vi "about GUI.vi"(8 "error in (no error)":errorcluster) -> (0 "error out":errorcluster)   [LabVIEW 2020, in "main.lvlib"]
uses:
  main.lvlib
  PTRL/GUI_tools/GUI_tools.lvlib
panel:
  out "about message":string
  in  "bottom_right":u32(colorbox)=16764108
  in  "top_left":u32(colorbox)=13434847
  # "Visible to user"
  # "Knight Tour"
  # "Resources\n1. https://en.wikipedia.org/wiki/Knight%27s_tour\n2. http://www.behnel.de/knight.html\n3. http://www.axel-conrad.de/springer/springer.html\n4. https://oeis.org/A165134 \n5. https://oeis.org/A165134/a165134.txt"
  # "Invisible to user"
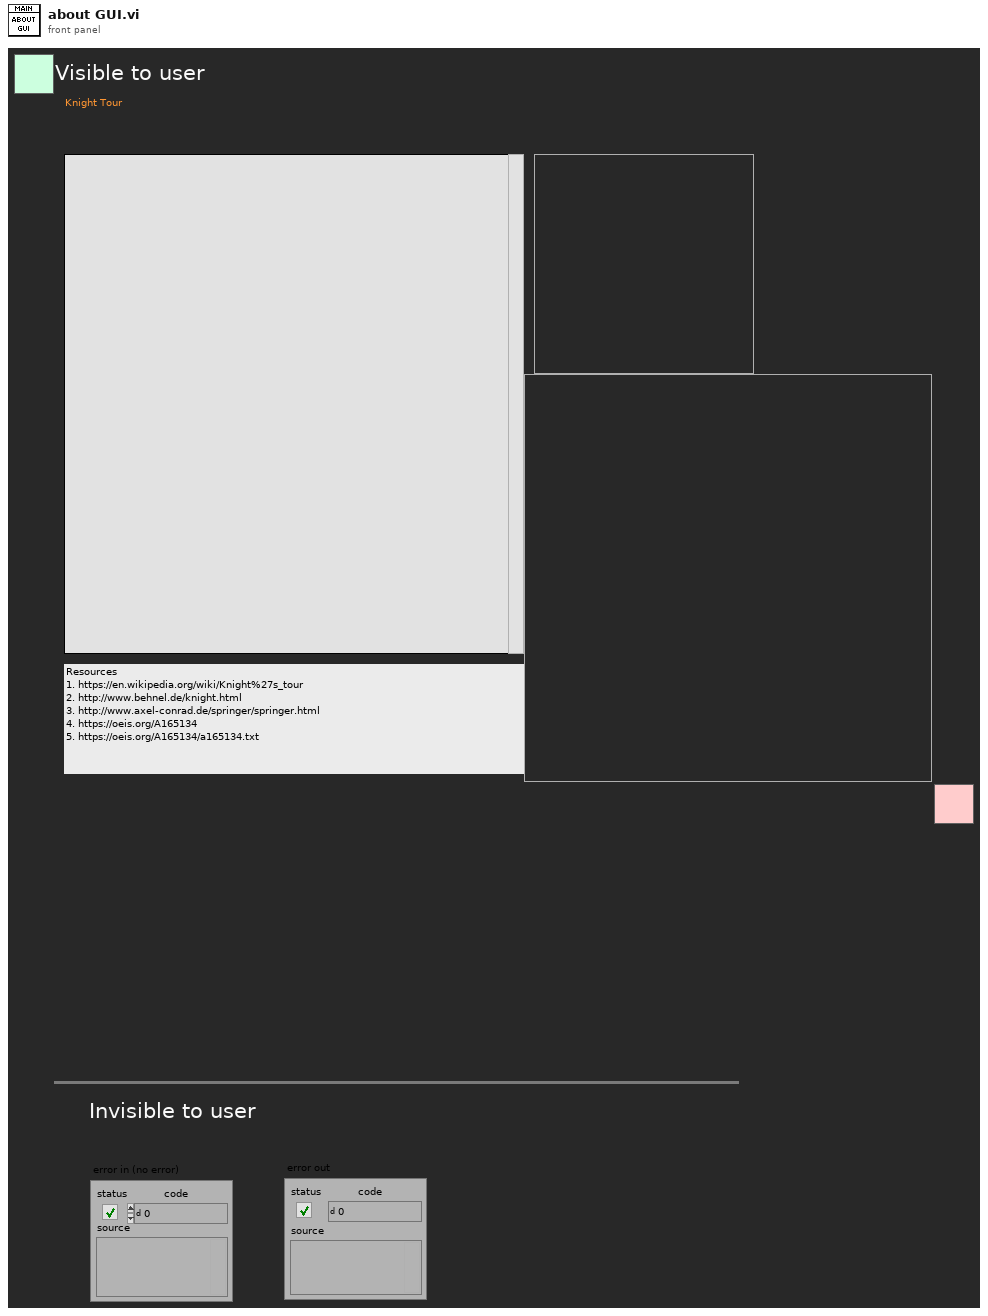
[diagram p1: front panel]
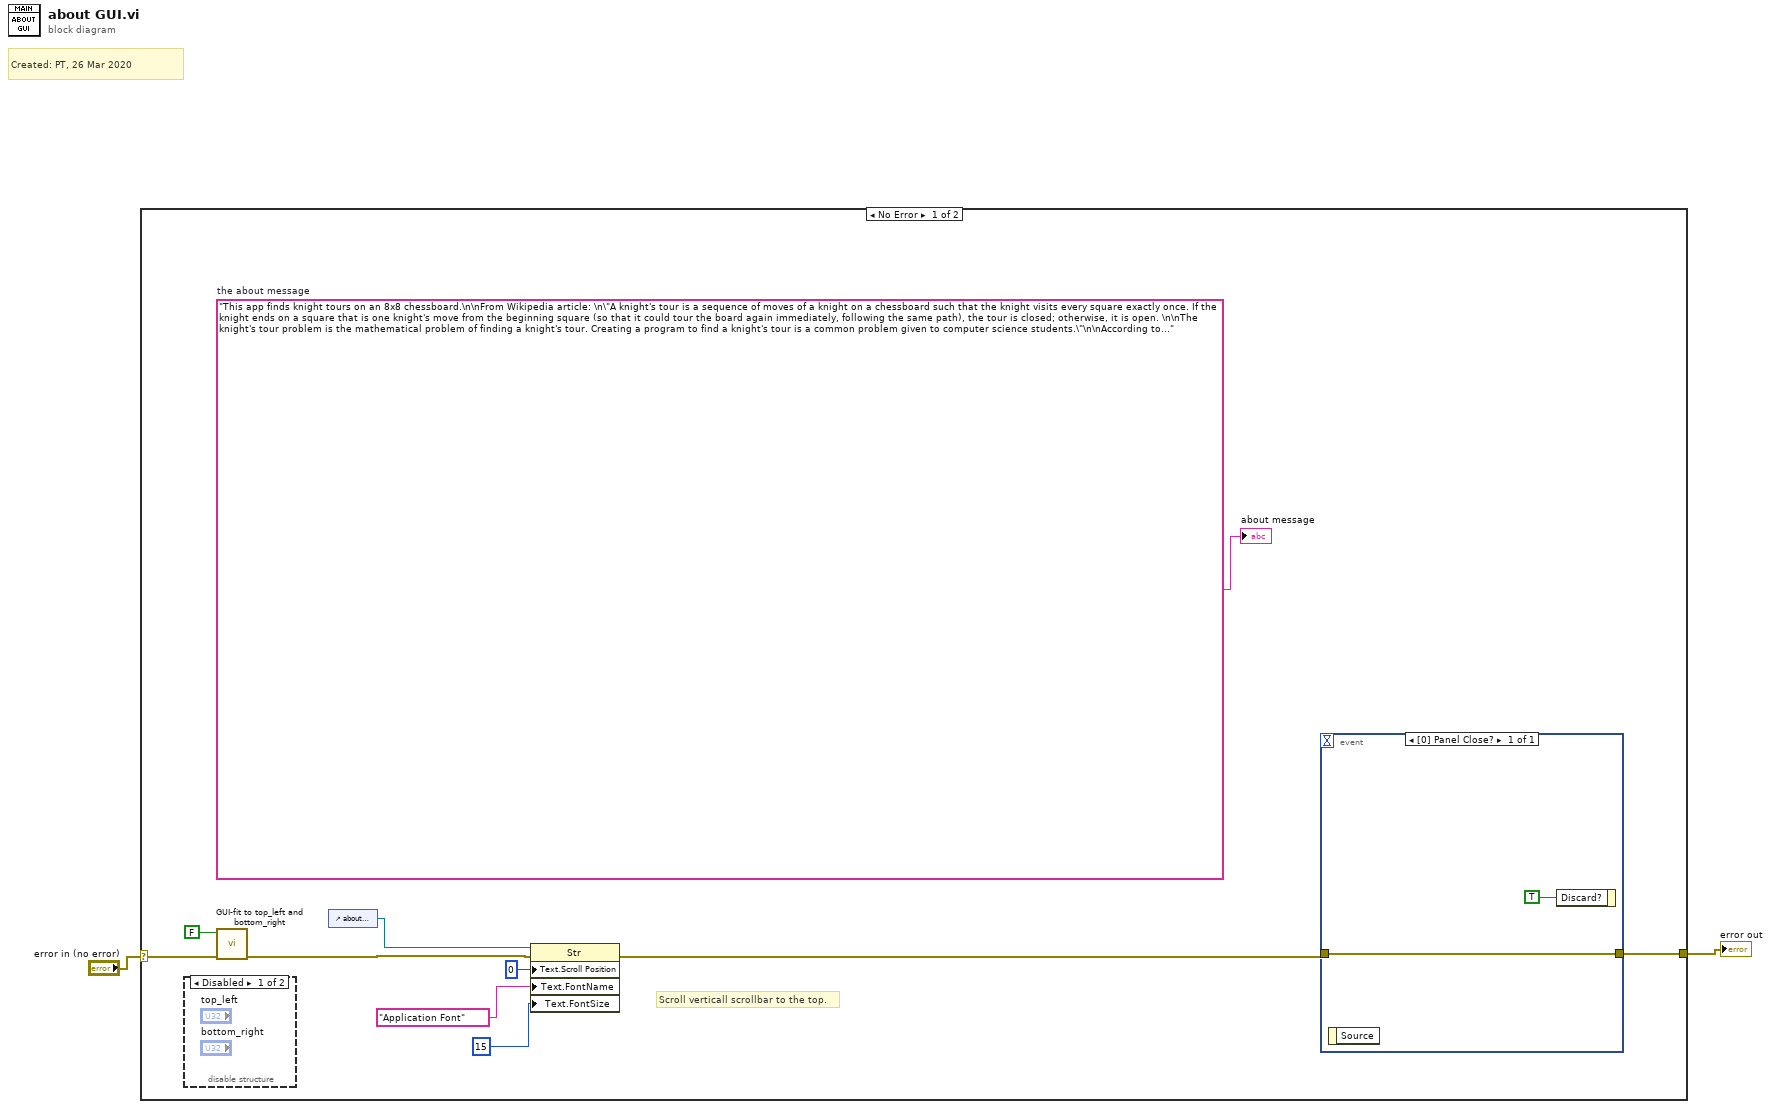
[diagram p0: block diagram]
diagram:
  # "Created: PT, 26 Mar 2020"
  n1 = case shown="No Error" "error in (no error)" {
    selector: "error in (no error)" -> [w11 w15]
    tunnel: [w12 w15] -> w2
    frame No Error {
      w10 = "This app finds knight tours on an 8x8 chessboard.\n\nFrom Wikipedia article: \n\"A knight's tour is a sequence of moves of a knight on a chessboard such that the knight visits every square exactly once. If the knight ends on a square that is one knight's move from the beginning square (so that it could tour the board again immediately, following the same path), the tour is closed; otherwise, it is open. \n\nThe knight's tour problem is the mathematical problem of finding a knight's tour. Creating a program to find a knight's tour is a common problem given to computer science students.\"\n\nAccording to Wikipedia, the total number of tours on an 8x8 chessboard is 19,591,828,170,979,904 (approx. 19.6 million billion tours) of which\n   o\t19,565,293,442,158,840 are open (99.86%)\n   o\t26,534,728,821,064 are closed (0.14 %)\n\nEven though the app finds tours fairly quickly, it cannot come close to finding all the tours (this had been my goal prior to reading the Wikipedia article).\n\nThe core of the app is a depth-first search (DFS) graph traversal, backtracking routine. The app uses Warnsdorff's rule to determine which square the knight should move to next: \"the knight is moved so that it always proceeds to the square from which the knight will have the fewest onward moves.\" (Wikipedia). When there is a tie (two or more potential next squares have the same smallest number of onwards moves) the app breaks the tie by selecting the first potential next square in trigonometric order (An angle can be drawn between each potential new square and the square the knight currently exists on. The app chooses the next square with the smallest angle).\n\nDue to following 1) Warndorff's rule and 2) a deterministic (non-random) tie-break system (trigonometric order selection), the app selects each next square in a predictable, deterministic way. Running the app twice produces the same tours in the same order. This is helpful because it enables the measurement of effects of changes to the core routine (e.g. performance optimisations).\n\nUse the controls in the tutorial section to slow down or pause the movement of the knight.\n\nThe app can display and log reports of each tour. The minimal format displays/logs the sequence of squares that form a tour. The detailed format displays/logs several other interesting pieces of information such as the time taken to find that tour and the total no. of moves forward and backward that were executed to find the tour.\n\nFuture desirable features:\n   o\tUser-selectable starting square. The starting square is currently hardcoded as a1.\n   o\tUser-selectable board size: 5x5, 6x6, 7x7, 8x8 or larger. Knight tours are not possible on 4x4 boards or smaller.\n\nApp written in LabVIEW 2018 64-bit.\n\nPT, 28 March 2020"  # the about message
      # "Scroll verticall scrollbar to the top."
      # "All good so far."
      n2 = disable-structure shown="Disabled" {
        frame Disabled {
        }
        frame Enabled {
        }
      }
      n3 = call "GUI-fit to top_left and bottom_right.vi"("error in (no error)"=w11, "Center Front Panel? (Dflt=T)"=FALSE) -> ("error out"=w9:errorcluster)  [unwired: 9 in]
      n4 = control-ref of="about message"() -> (w7:refnum<vi>)
      n5 = property class="Str"(reference=w7, error in=w9, "Text.Scroll Position"=u32 0, "Text.FontName"="Application Font", "Text.FontSize"=u32 15 ("Text.Font:Size")) -> (error out=w8:errorcluster)  [unwired: 1 out]
      n6 = event shown="[0] Panel Close?" {
        selector: _ -> [_]
        dyn-events: _ -> [_]
        timeout: _ -> [_]
        tunnel: w8 -> [w14]
        tunnel: [w14] -> w12
        event Panel Close? {
          n7 = event-data() -> ()  [unwired: 1 in, 1 out]
          n8 = event-data("Discard?"=TRUE) -> ()  [unwired: 1 in, 1 out]
        }
      }
      "about message" <- w10
    }
    frame Error {
    }
  }
  "error out" <- w2
